vi "list call cond.vi"(8 "error in (no error)":errorcluster, 9 "position":i32, 10 "mask_0":u16, 11 "mask_1":u16) -> (0 "error out":errorcluster)   [LabVIEW 2015, in "SCANalone4x64.lvlib"]
doc: "__declspec(dllimport) void __stdcall list_call_cond(unsigned short mask_1, unsigned short mask_0, long position);"
uses:
  <userlib>/SCANalone4x64/SCANalone4x64.lvlib
  <userlib>/SCANalone4x64/SCANalone4x64.dll
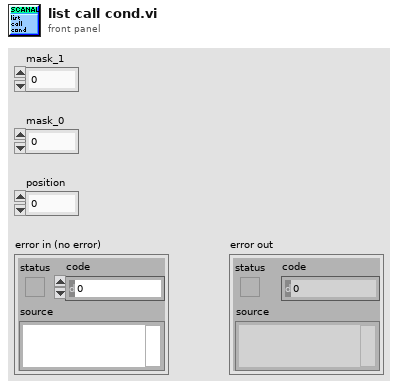
[diagram p1: front panel]
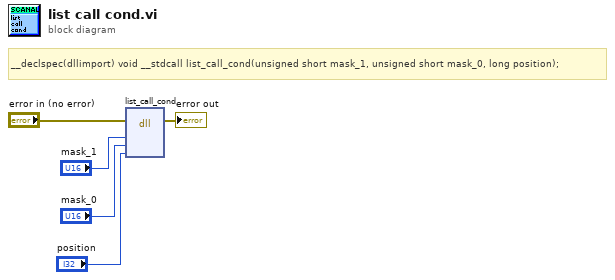
[diagram p0: block diagram]
diagram:
  # "__declspec(dllimport) void __stdcall list_call_cond(unsigned short mask_1, unsigned short mask_0, long position);"
  n1 = dll-call lib="C:/Program Files/National Instruments/LabVIEW 2015/user.lib/SCANalone4x64/SCANalone4x64.*" fn="list_call_cond"(error in="error in (no error)", "mask_1"="mask_1", "mask_0"="mask_0", "position"="position") -> (error out=→"error out":errorcluster)  [unwired: 6 in, 1 out]
